vi "test -- linear regression.vi"() -> ()   [LabVIEW 2021]
uses:
  array -- bilinear regression 2D.ctl
  4-vec-array.ctl
  array -- fit control .ctl
  <vilib>/Analysis/baseanly.llb/Mean (DBL).vi
  <vilib>/Analysis/7linalg.llb/Solve Linear Equations.vi
  <vilib>/Analysis/7linalg.llb/Solve Linear Equations (single right hand).vi
  <vilib>/Analysis/baseanly.llb/A x B.vi
  <vilib>/Analysis/baseanly.llb/Real A x B.vi
  <vilib>/Analysis/baseanly.llb/Solve Linear Equations By Cholesky.vi
  <vilib>/Analysis/baseanly.llb/Real Matrix to Compact Array.vi
  <vilib>/Analysis/baseanly.llb/Real Compact Tri-Matrix Linear Eqs.vi
  <vilib>/Analysis/Matrix/Numeric/Conversions/Array To Matrix.vi
  <vilib>/Analysis/Matrix/Numeric/Conversions/Array To Matrix - RA2.vi
  <vilib>/Analysis/7linalg.llb/Solve Linear Eqs (General).vi
  <vilib>/Analysis/7linalg.llb/Solve Linear Eqs (Gen, single right hand).vi
  <vilib>/Analysis/Matrix/Numeric/Subtract/Subtract.vi
  <vilib>/Analysis/Matrix/Numeric/Subtract/Subtract - RM,RM.vi
  <vilib>/Analysis/Matrix/Numeric/Conversions/Matrix To Array.vi
  <vilib>/Analysis/Matrix/Numeric/Conversions/Matrix To Array - RM.vi
  <vilib>/Analysis/NI_AALBase.lvlib
panel:
  in  "noise factor":dbl=0.1 format="%#_13g"
  out "linear fit map out":map{T1, dbl}(c390)
  out "xyzw IN bilinear out":T2={"x"=[-2.0, -1.0, 0.0, 1.0, 2.0], "y"=[-2.0, -1.0, 0.0, 1.0, 2.0], "w"=[-2.0, -1.0, 0.0, 1.0, 2.0], "z"=[12.0, 3.0, 0.0, 3.0, 12.0]}
  out "xyzw out sum of two":T2={"x"=[-2.0, -1.0, 0.0, 1.0, 2.0], "y"=[-2.0, -1.0, 0.0, 1.0, 2.0], "w"=[-2.0, -1.0, 0.0, 1.0, 2.0], "z"=[12.0, 3.0, 0.0, 3.0, 12.0]}
  out "fit map out bilinear":map{T1, dbl}(c390)
  in  "axx\naxy\nayy\nbx\nby\nc \nbilinear":T1[][](array[typedef])=[[enum."xx"], [enum."yy"], [enum."ww"], [enum."yw"], [enum."xw"], [enum."xy"], [enum."x"], [enum."y"], [enum."w"], [enum."1"]]
  in  "bilinear   IN":dbl[](array[numeric])=[1.0, 1.0, 1.0, 1.0, 0.0, 0.0, 0.0, 0.0, 0.0, 0.0]
  out "xyzw linear out":T2={"x"=[-2.0, -1.0, 0.0, 1.0, 2.0], "y"=[-2.0, -1.0, 0.0, 1.0, 2.0], "w"=[-2.0, -1.0, 0.0, 1.0, 2.0], "z"=[12.0, 3.0, 0.0, 3.0, 12.0]}
  in  "axx\naxy\nayy\nbx\nby\nc":T1[][](array[typedef])=[[enum."x"], [enum."y"], [enum."w"], [enum."1"]]
  in  "linear  IN":dbl[](array[numeric])=[1.0, 1.0, 1.0, 1.0]
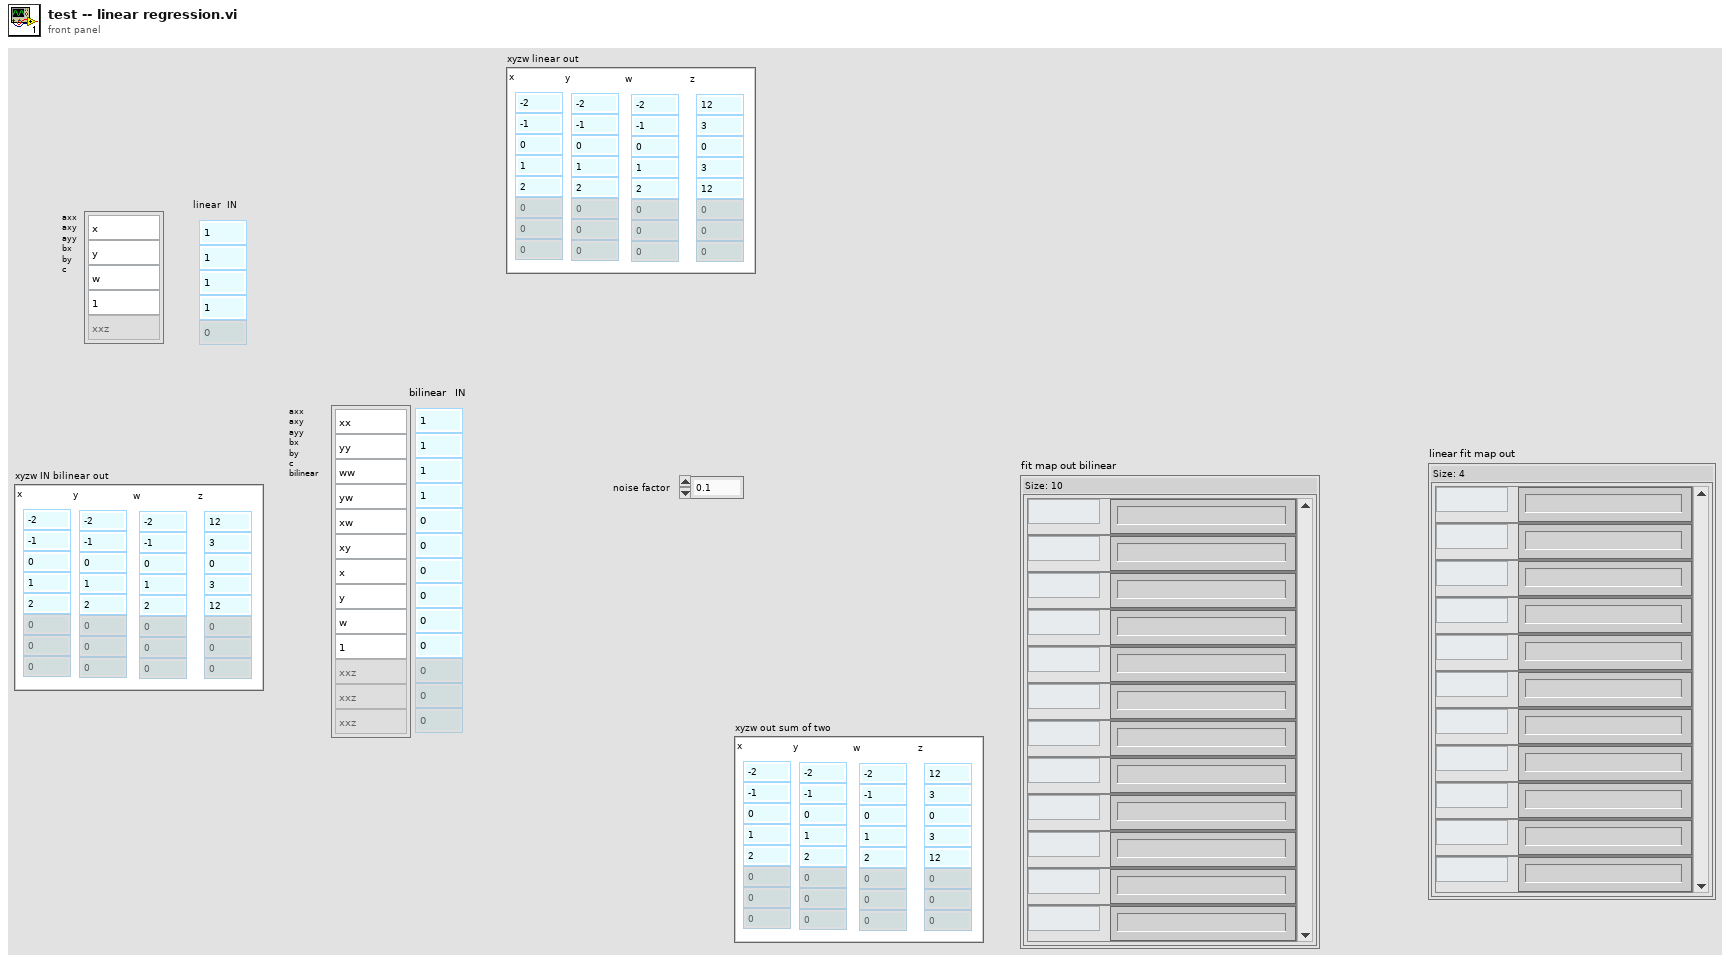
[diagram p1: front panel]
types:
  T1 = typedef "array -- bilinear regression 2D.ctl" = enum16{"1", "x", "y", "xx", "xy", "yy", "xxy", "xyy", "yyy", "xxx", "xxyy", "xyyy", "xxxy", "yyyy", "xxxx", "xxz", "xyz", "yyz", "xz", "yz", "z", "wwz", "ywz", "xwz", "xxxw", "xxyw", "xyyw", "yyyw", "xxww", "xyww", "yyww", "xwww", "ywww", "wwww", "ww", "xw", "yw", "w", "wz", "xxw", "yyw", "xyw", "xww", "yww", "www"}
  T2 = typedef "4-vec-array.ctl" = cluster{"x":dbl[], "y":dbl[], "w":dbl[], "z":dbl[]}
  T3 = typedef "array -- fit control .ctl" = enum16{"fit", "calc", "check", "init"}
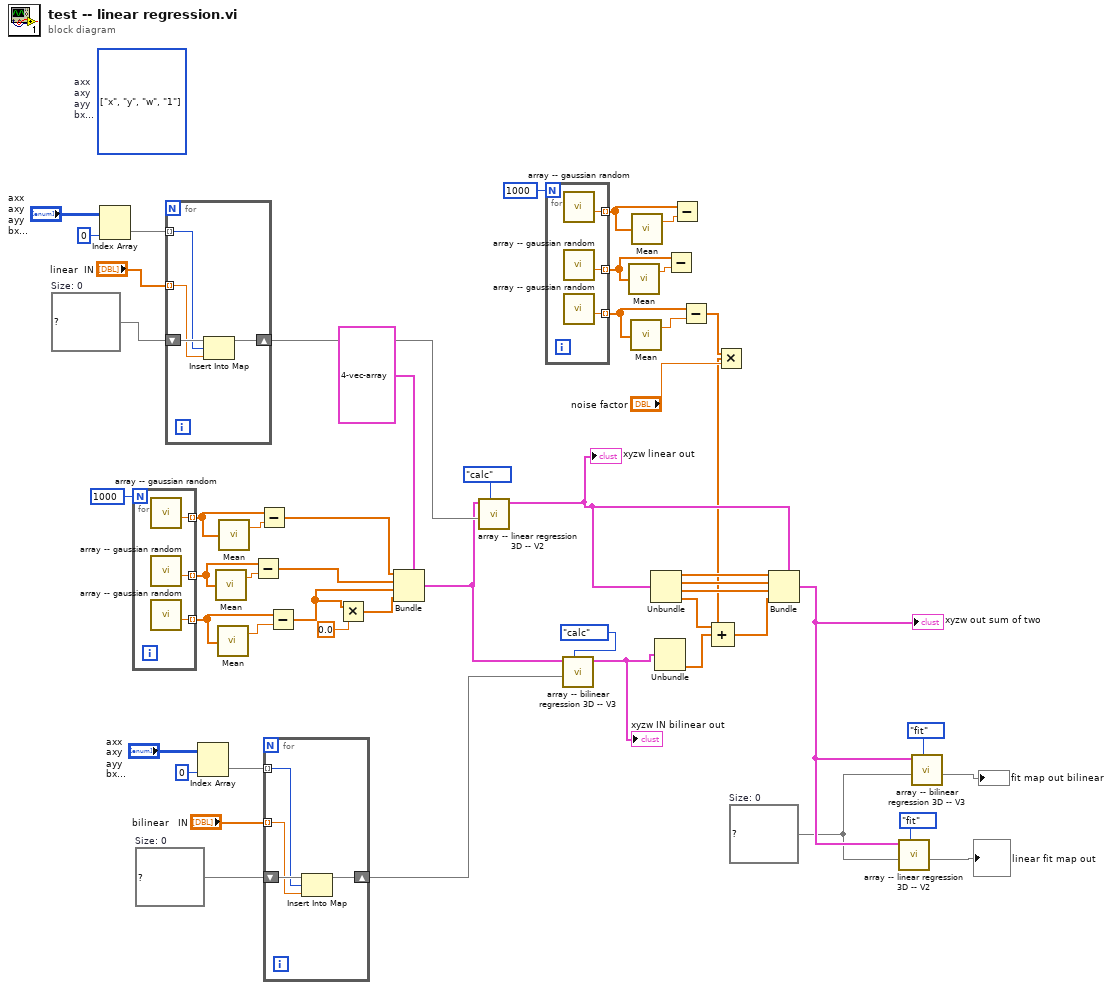
[diagram p0: block diagram]
diagram:
  w15 = map{T1, dbl} {}  # Size: 0
  w40 = map{T1, dbl} {}  # Size: 0
  w47 = map{T1, dbl} {}  # Size: 0
  (unwired) T1[][] [[enum."x"], [enum."y"], [enum."w"], [enum."1"]] items=["1", "x", "y", "xx", "xy", "yy", "xxy", "xyy", "yyy", "xxx", "xxyy", "xyyy", "xxxy", "yyyy", "xxxx", "xxz", "xyz", "yyz", "xz", "yz", "z", "wwz", "ywz", "xwz", "xxxw", "xxyw", "xyyw", "yyyw", "xxww", "xyww", "yyww", "xwww", "ywww", "wwww", "ww", "xw", "yw", "w", "wz", "xxw", "yyw", "xyw", "xww", "yww", "www"]  # axx axy ayy bx by c
  n1 = Index Array(array="axx\naxy\nayy\nbx\nby\nc", index (col)=0 ("disabled index (col)")) -> (element=w49:T1[])  [unwired: 1 in]
  n2 = for {
    N: 1000 -> [_]
    tunnel: [w55] -> w29 mode=indexing
    tunnel: [w54] -> w26 mode=indexing
    tunnel: [w53] -> w27 mode=indexing
    n3 = call "array -- gaussian random.vi"() -> ("number"=w55:dbl)  [unwired: 11 in]
    n4 = call "array -- gaussian random.vi"() -> ("number"=w54:dbl)  [unwired: 11 in]
    n5 = call "array -- gaussian random.vi"() -> ("number"=w53:dbl)  [unwired: 11 in]
  }
  n6 = for {
    tunnel: w49 -> [w57] mode=indexing
    tunnel: "linear  IN" -> [w58] mode=indexing
    shift-right: [w56] -> w46
    shift-left: w47 -> [w59]
    n7 = Insert Into Map(map in=w59, key=w57, value=w58) -> (map out=w56:map{T1, dbl})  [unwired: 2 out]
  }
  n8 = Index Array(array="axx\naxy\nayy\nbx\nby\nc \nbilinear", index (col)=0 ("disabled index (col)")) -> (element=w42:T1[])  [unwired: 1 in]
  n9 = call-poly <vilib>:"Mean.vi"("X"=w26) -> ("mean"=w25:dbl)  [unwired: 1 out]
  n10 = call-poly <vilib>:"Mean.vi"("X"=w27) -> ("mean"=w28:dbl)  [unwired: 1 out]
  n11 = call-poly <vilib>:"Mean.vi"("X"=w29) -> ("mean"=w30:dbl)  [unwired: 1 out]
  n12 = Subtract(x=w26, y=w25) -> (x-y=w23:dbl[])
  n13 = Subtract(x=w29, y=w30) -> (x-y=w24:dbl[])
  n14 = for {
    tunnel: w42 -> [w61] mode=indexing
    tunnel: "bilinear   IN" -> [w62] mode=indexing
    shift-right: [w60] -> w39
    shift-left: w40 -> [w63]
    n15 = Insert Into Map(map in=w63, key=w61, value=w62) -> (map out=w60:map{T1, dbl})  [unwired: 2 out]
  }
  n16 = Subtract(x=w27, y=w28) -> (x-y=w14:dbl[])
  n17 = Multiply(x=w14, y=0.0) -> (x*y=w13:dbl[])
  n18 = Bundle(cluster=T2 {"x"=array[1000 elements], "y"=array[1000 elements], "w"=array[1000 elements], "z"=array[1000 elements]} ("xyzw IN bilinear out 2"), "x"=w24, "y"=w23, "w"=w14, "z"=w13) -> (w18:T2)
  n19 = call "array -- linear regression 3D -- V2.vi"("action"=array_--_fit_control_."calc", "fit map IN"=w46, "xyzw IN"=w18) -> ("xyzw OUT"=w38:T2)  [unwired: 7 in, 1 out]
  "xyzw linear out" <- w38
  n20 = for {
    N: 1000 -> [_]
    tunnel: [w66] -> w8 mode=indexing
    tunnel: [w65] -> w5 mode=indexing
    tunnel: [w64] -> w6 mode=indexing
    n21 = call "array -- gaussian random.vi"() -> ("number"=w66:dbl)  [unwired: 11 in]
    n22 = call "array -- gaussian random.vi"() -> ("number"=w65:dbl)  [unwired: 11 in]
    n23 = call "array -- gaussian random.vi"() -> ("number"=w64:dbl)  [unwired: 11 in]
  }
  n24 = call "array -- bilinear regression 3D -- V3.vi"("action"=array_--_fit_control_."calc", "fit map IN"=w39, "xyzw IN"=w18) -> ("xyzw OUT"=w16:T2)  [unwired: 7 in, 1 out]
  "xyzw IN bilinear out" <- w16
  n25 = call-poly <vilib>:"Mean.vi"("X"=w5) -> ("mean"=w4:dbl)  [unwired: 1 out]
  n26 = call-poly <vilib>:"Mean.vi"("X"=w6) -> ("mean"=w7:dbl)  [unwired: 1 out]
  n27 = call-poly <vilib>:"Mean.vi"("X"=w8) -> ("mean"=w9:dbl)  [unwired: 1 out]
  n28 = Unbundle(w38) -> ("x"=w34:dbl[], "y"=w33:dbl[], "w"=w32:dbl[], "z"=w37:dbl[])
  n29 = Unbundle(w16) -> ("z"=w35:dbl[])  [unwired: 3 out]
  n30 = Subtract(x=w5, y=w4) -> ()  [unwired: 1 out]
  n31 = Subtract(x=w8, y=w9) -> ()  [unwired: 1 out]
  n32 = Subtract(x=w6, y=w7) -> (x-y=w2:dbl[])
  n33 = Multiply(x=w2, y="noise factor") -> (x*y=w1:dbl[])
  n34 = Compound Arithmetic op=ADD(w37, w35, w1) -> (w36:dbl[])
  n35 = Bundle(cluster=w38, "x"=w34, "y"=w33, "w"=w32, "z"=w36) -> (w17:T2)
  "xyzw out sum of two" <- w17
  n36 = call "array -- linear regression 3D -- V2.vi"("action"=array_--_fit_control_."fit", "fit map IN"=w15, "xyzw IN"=w17) -> ("fit map out"=→"linear fit map out":map{T1, dbl})  [unwired: 7 in, 1 out]
  n37 = call "array -- bilinear regression 3D -- V3.vi"("action"=array_--_fit_control_."fit", "fit map IN"=w15, "xyzw IN"=w17) -> ("fit map out"=→"fit map out bilinear":map{T1, dbl})  [unwired: 7 in, 1 out]
